vi "unitcontour2array.vi"(11 "unit contour":T1) -> (3 "Array":dbl[][](array[numeric]))   [LabVIEW 2017]
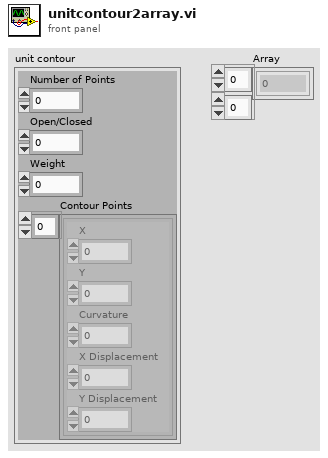
[diagram p1: front panel]
types:
  T1 = cluster{"Number of Points":i32, "Open/Closed":i32, "Weight":dbl, "Contour Points":cluster{"X":dbl, "Y":dbl, "Curvature":dbl, "X Displacement":dbl, "Y Displacement":dbl}[]}
  T2 = cluster{"X":dbl, "Y":dbl, "Curvature":dbl, "X Displacement":dbl, "Y Displacement":dbl}[]
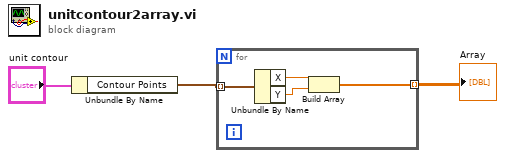
[diagram p0: block diagram]
diagram:
  n1 = Unbundle By Name("unit contour") -> ("Contour Points"=w2:T2)
  n2 = for {
    tunnel: w2 -> [w7] mode=indexing
    tunnel: [w4] -> w3 mode=indexing
    n3 = Unbundle By Name(w7) -> ("X"=w6:dbl, "Y"=w5:dbl)
    n4 = Build Array(w6, w5) -> (w4:dbl[])
  }
  "Array" <- w3
